vi "USB Open.vi"(8 "error in (no error)":errorcluster, 11 "Device ID":i32) -> (0 "error out":errorcluster, 2 "Return Code":i32, 3 "Device ID out":i32)   [LabVIEW 2014, in "Keyence LJ-V7000.lvlib"]
uses:
  Keyence LJ-V7000.lvlib
panel:
  # "(c) 2012 KEYENCE CORPORATION.  ALL RIGHTS RESERVED."
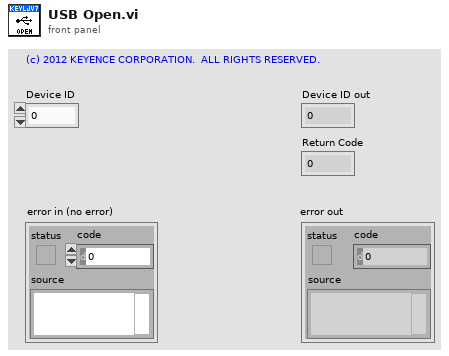
[diagram p1: front panel]
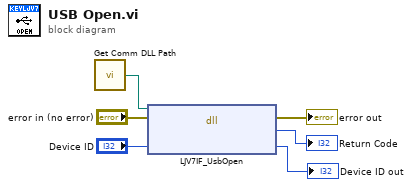
[diagram p0: block diagram]
diagram:
  n1 = call "Get Comm DLL Path.vi"() -> ("Comm DLL Path"=w1:path)  [unwired: 1 in]
  n2 = dll-call lib="C:/Program Files/National Instruments/LabVIEW 2011/instr.lib/Keynece LJ-V7000/LJV7_IF.*" fn="LJV7IF_UsbOpen"(path in=w1, error in="error in (no error)", "lDeviceId"="Device ID") -> (error out=→"error out":errorcluster, "lRetCode"=→"Return Code":i32, "lDeviceId"=→"Device ID out":i32)  [unwired: 1 in, 1 out]
